vi "QueueDriver.vi"(0 "Queue Name":string, 5 "State":string, 7 "State  s[]":string[](array[string]), 11 "error in (no error)":errorcluster, 13 "Operation":T1) -> (4 "Dequeued Element":string, 15 "error out":errorcluster)   [LabVIEW 2020]
uses:
  Controls/QueueOperations.ctl
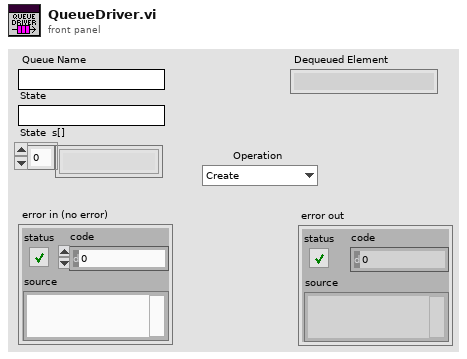
[diagram p1: front panel]
types:
  T1 = typedef "QueueOperations.ctl" = enum16{"Create", "Enqueue", "Enqueue N", "Enstack", "Dequeue", "Flush", "Release"}
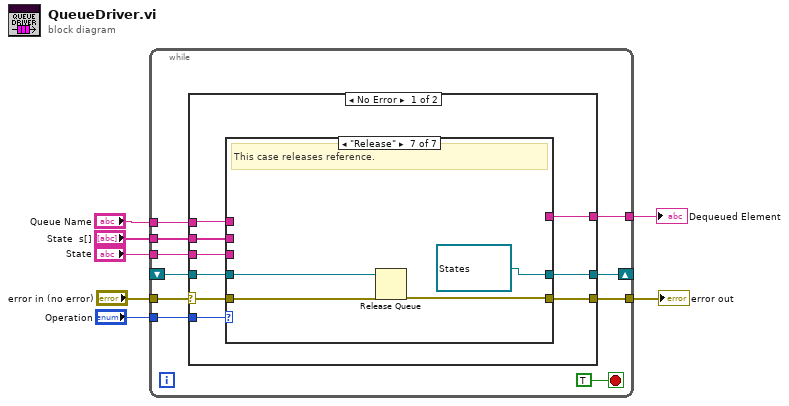
[diagram p0: block diagram]
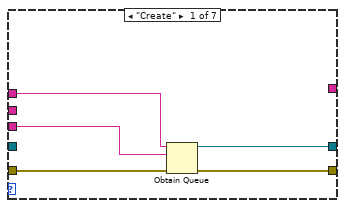
[diagram p2: hidden frame]
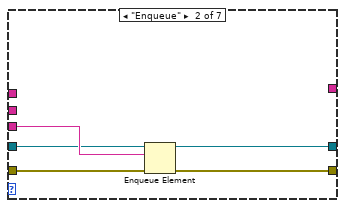
[diagram p3: hidden frame]
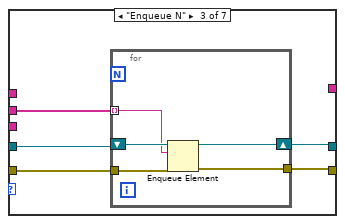
[diagram p4: hidden frame]
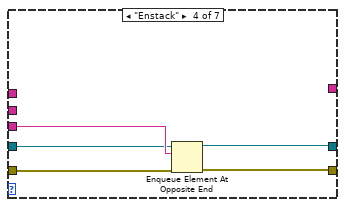
[diagram p5: hidden frame]
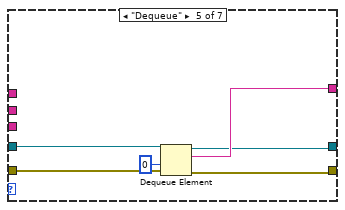
[diagram p6: hidden frame]
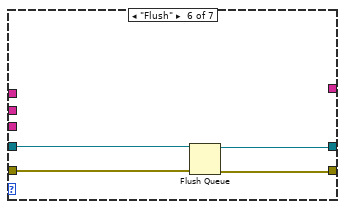
[diagram p7: hidden frame]
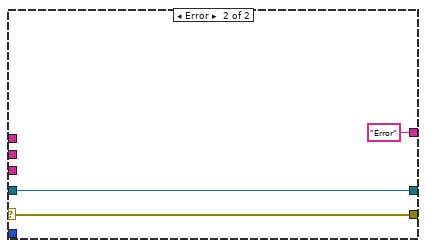
[diagram p8: hidden frame]
diagram:
  n1 = while {
    tunnel: "error in (no error)" -> [w17]
    tunnel: "Queue Name" -> [w16]
    tunnel: [w15] -> w3
    tunnel: "State" -> [w14]
    shift-right: [w13] -> _
    shift-left: _ -> [w12]
    tunnel: [w11] -> w4
    tunnel: "State  s[]" -> [w9]
    tunnel: "Operation" -> [w8]
    stop <- TRUE stop-if-true
    n2 = case shown="No Error" w17 {
      selector: w17 -> [w25 w67]
      tunnel: w16 -> [w26 _]
      tunnel: [w24 w67] -> w15
      tunnel: w14 -> [w23 _]
      tunnel: [w22 w68] -> w13
      tunnel: w12 -> [w21 w68]
      tunnel: [w20 "Error" ("States")] -> w11
      tunnel: w9 -> [w19 _]
      tunnel: w8 -> [w18 _]
      frame No Error {
        n3 = case shown="\"Release\"" w18 {
          tunnel: w26 -> [w31 _ _ _ _ _ _]
          tunnel: w25 -> [w30 w36 w41 w51 w57 w61 w65]
          tunnel: [w27 w32 w40 w47 w53 w58 w64] -> w24
          tunnel: w23 -> [w29 w35 _ w50 _ _ _]
          tunnel: [w28 w34 w38 w49 w54 w59 refnum<queue> refnum ("queue out")] -> w22
          tunnel: w21 -> [_ w33 w39 w48 w55 w60 w63]
          tunnel: [_ _ _ _ w56 _ _] -> w20
          tunnel: w19 -> [_ _ w37 _ _ _ _]
          frame "Create" {
            n4 = Obtain Queue(name (unnamed)=w31, element data type=w29, error in (no error)=w30) -> (queue out=w28:refnum<queue>, error out=w27:errorcluster)  [unwired: 2 in, 1 out]
          }
          frame "Enqueue" {
            n5 = Enqueue Element(queue=w33, element=w35, error in (no error)=w36) -> (queue out=w34:refnum<queue>, error out=w32:errorcluster)  [unwired: 1 in, 1 out]
          }
          frame "Enqueue N" {
            n6 = for {
              tunnel: w41 -> [w46]
              tunnel: [w45] -> w40
              shift-right: [w43] -> w38
              shift-left: w39 -> [w44]
              tunnel: w37 -> [w42] mode=indexing
              n7 = Enqueue Element(queue=w44, element=w42, error in (no error)=w46) -> (queue out=w43:refnum<queue>, error out=w45:errorcluster)  [unwired: 1 in, 1 out]
            }
          }
          frame "Enstack" {
            n8 = Enqueue Element At Opposite End(queue=w48, element=w50, error in (no error)=w51) -> (queue out=w49:refnum<queue>, error out=w47:errorcluster)  [unwired: 1 in, 1 out]
          }
          frame "Dequeue" {
            n9 = Dequeue Element(queue=w55, timeout in ms (-1)=0, error in (no error)=w57) -> (queue out=w54:refnum<queue>, element=w56:string, error out=w53:errorcluster)  [unwired: 1 out]
          }
          frame "Flush" {
            n10 = Flush Queue(queue=w60, error in (no error)=w61) -> (queue out=w59:refnum<queue>, error out=w58:errorcluster)  [unwired: 1 out]
          }
          frame "Release" {
            # "This case releases reference."
            n11 = Release Queue(queue=w63, error in (no error)=w65) -> (error out=w64:errorcluster)  [unwired: 1 in, 2 out]
          }
        }
      }
      frame Error {
      }
    }
  }
  "error out" <- w3
  "Dequeued Element" <- w4
